vi "Send Discovery Payload.vi"(8 "error in (no error)":errorcluster, 11 "DiscoveryService in":refnum<class "NodeDiscovery.lvclass">) -> (0 "error out":errorcluster, 3 "DiscoveryService out":refnum<class "NodeDiscovery.lvclass">)   [LabVIEW 2020, in "Vecto.lvlib" / "NodeDiscovery.lvclass"]
uses:
  NodeDiscovery.lvclass
  NodeDiscovery.lvclass/NodeDiscovery.ctl
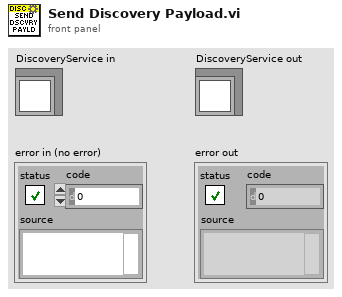
[diagram p1: front panel]
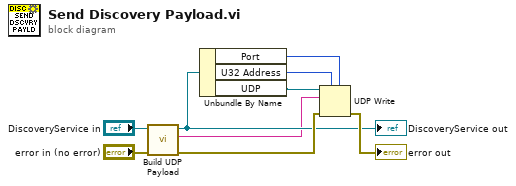
[diagram p0: block diagram]
diagram:
  n1 = call "Build UDP Payload.vi"("error in (no error)"="error in (no error)", "DiscoveryService in"="DiscoveryService in") -> ("error out"=w3:errorcluster, "UDP Payload"=w1:string, "DiscoveryService out"=w2:refnum<class "NodeDiscovery.lvclass">)  [unwired: 7 in]
  "DiscoveryService out" <- w2
  n2 = Unbundle By Name(w2) -> ("Port"=w5:u16, "U32 Address"=w7:u32, "UDP"=w6:refnum<k16>)
  n3 = UDP Write(address=w7, port or service name=w5, connection ID=w6, data in=w1, 8:w3) -> (error out=→"error out":errorcluster)  [unwired: 1 in, 1 out]
